vi "Startsequenz.vi"(11 "NXT":T1={"error"={"status"=FALSE, "code"=0, "source"=""}, "address"="", "NXT #"=-1, "Show Error"=TRUE, "Connection"=4} {"Connection" items=["USB", "Bluetooth", "USB then Bluetooth", "Last Connection", "Preference"]}) -> (3 "NXT 2":T1={"error"={"status"=FALSE, "code"=0, "source"=""}, "address"="", "NXT #"=-1, "Show Error"=TRUE, "Connection"=4} {"Connection" items=["USB", "Bluetooth", "USB then Bluetooth", "Last Connection", "Preference"]})   [LabVIEW 2009]
uses:
  <vilib>/NXT/Subs/LVHSConnector.ctl
  <vilib>/NXT/Subs/MotorOutput.ctl
  <vilib>/NXT/Dual Mode Library/Waits/Wait_Num(msec).vi
  <vilib>/NXT/Dual Mode Library/Motors/ResetMotor.vi
  <vilib>/NXT/Dual Mode Library/Display/drawText.vi
  <vilib>/NXT/Dual Mode Library/Display/clearDisplay.vi
  <vilib>/NXT/Dual Mode Library/Sound/Tone.vi
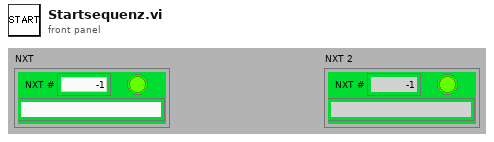
[diagram p1: front panel]
types:
  T1 = typedef "LVHSConnector.ctl" = cluster{"error":errorcluster, "address":string, "NXT #":i32, "Show Error":bool, "Connection":u16}
  T2 = typedef "MotorOutput.ctl" = u8
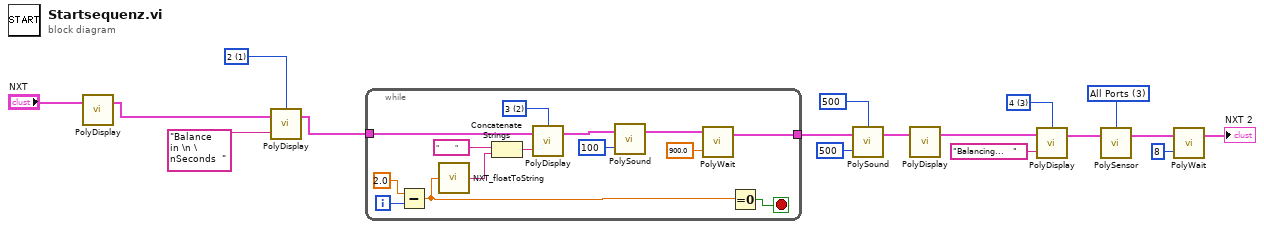
[diagram p0: block diagram]
diagram:
  w6 = T2 3 items=["Port A", "Port B", "Port C", "All Ports"] ("Port (All Ports)")
  w8 = i16 3 items=["1", "2", "3", "4", "5", "6", "7", "8"] ("Line")
  w16 = i16 1 items=["1", "2", "3", "4", "5", "6", "7", "8"] ("Line")
  n1 = call-poly <vilib>:"PolyDisplay.vi"("NXT"="NXT") -> ("NXT"=w10:T1)  [unwired: 3 in]
  n2 = call-poly <vilib>:"PolyDisplay.vi"("Text"="Balance in \n \nSeconds  ", "NXT"=w10, "Line"=w16) -> ("NXT"=w15:T1)  [unwired: 1 in]
  n3 = while {
    tunnel: w15 -> [w22]
    tunnel: [w21] -> w14
    i -> [w28]
    stop <- w27 stop-if-true
    w30 = i16 2 items=["1", "2", "3", "4", "5", "6", "7", "8"] ("Line")
    n4 = Subtract(x=2.0, y=w28) -> (x-y=w26:dbl)
    n5 = call <vilib>:"NXT_floatToString.vi"("number"=w26) -> ("string"=w19:string)
    n6 = Concatenate Strings("        ", w19) -> (w20:string)
    n7 = call-poly <vilib>:"PolyDisplay.vi"("Text"=w20, "NXT"=w22, "Line"=w30) -> ("NXT"=w31:T1)  [unwired: 1 in]
    n8 = call-poly <vilib>:"PolySound.vi"("Duration (500 ms)"=u16 100, "NXT"=w31) -> ("NXT"=w24:T1)  [unwired: 2 in]
    n9 = call-poly <vilib>:"PolyWait.vi"("Time (100 msec)"=sgl 900.0 ("Time (1 sec)"), "NXT"=w24) -> ("NXT"=w21:T1)  [unwired: 2 in]
    n10 = Equal To 0?(x=w26) -> (x = 0?=w27:bool)
  }
  n11 = call-poly <vilib>:"PolySound.vi"("Duration (500 ms)"=u16 500, "NXT"=w14, "Tone (440 Hz)"=u16 500) -> ("NXT"=w5:T1)  [unwired: 1 in]
  n12 = call-poly <vilib>:"PolyDisplay.vi"("NXT"=w5) -> ("NXT"=w4:T1)  [unwired: 3 in]
  n13 = call-poly <vilib>:"PolyDisplay.vi"("Text"="Balancing...   ", "NXT"=w4, "Line"=w8) -> ("NXT"=w7:T1)  [unwired: 1 in]
  n14 = call-poly <vilib>:"PolySensor.vi"("NXT"=w7, "Port (All Ports)"=w6) -> ("NXT"=w2:T1)  [unwired: 2 in]
  n15 = call-poly <vilib>:"PolyWait.vi"("Time (100 msec)"=u32 8 ("Time (msec)"), "NXT"=w2) -> ("NXT"=→"NXT 2":T1)  [unwired: 2 in]
